vi "WPI_AccumulatorSetConfiguration.vi"(6 "Deadband":dbl, 8 "error in (no error)":errorcluster, 9 "Initial Value":dbl, 10 "Center":dbl, 11 "AIDeviceRef":T1={"DevStatus"={"status"=FALSE, "code"=0, "source"=""}, "Analog Channel"=enum."Invalid"}) -> (0 "error out":errorcluster, 3 "AIDeviceRef":T1={"DevStatus"={"status"=FALSE, "code"=0, "source"=""}, "Analog Channel"=enum."Invalid"})   [LabVIEW 2017]
doc: "Sets the center value, initial value, and deadband of the accumulator on the FPGA on the roboRIO device. The FPGA subtracts the center value from the value of each element before adding the value of the element to the cumulative value of the accumulator. Set the center value and initial value to account for offset in devices, such as gyros and accelerometers, when integrating signals from these devices. The accumulator does not accumulate a value if the difference between the center value and the current value is less than the deadband.\n\nThis software is licensed. Open the labview\\readme\\WPI Robotics Library Open Source License.txt file for more information."
uses:
  <vilib>/Rock Robotics/WPI/AnalogChannel/WPI_AnalogChannelDevRef.ctl
  <vilib>/Rock Robotics/SystemInterfaces/AI/FPGA_AIChannel.ctl
  <vilib>/Rock Robotics/SystemInterfaces/System/FPGA_SystemGet.vi
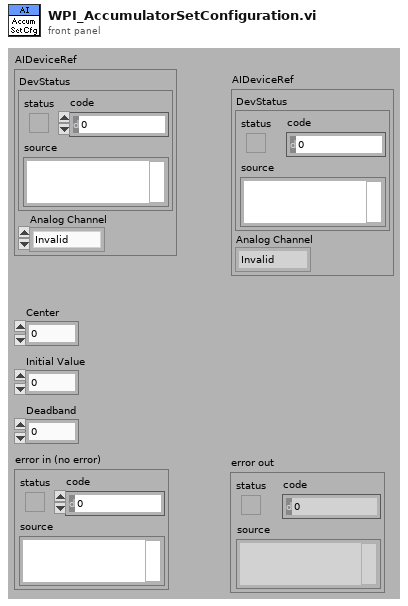
[diagram p1: front panel]
types:
  T1 = typedef "WPI_AnalogChannelDevRef.ctl" = cluster{"DevStatus":errorcluster, "Analog Channel":T2}
  T2 = typedef "FPGA_AIChannel.ctl" = enum8{"AI 0", "AI 1", "AI 2", "AI 3", "AI MXP 0", "AI MXP 1", "AI MXP 2", "AI MXP 3", "Invalid"}
  T3 = typedef "FPGA_AIDevRef.ctl" = cluster{"DevStatus":errorcluster}
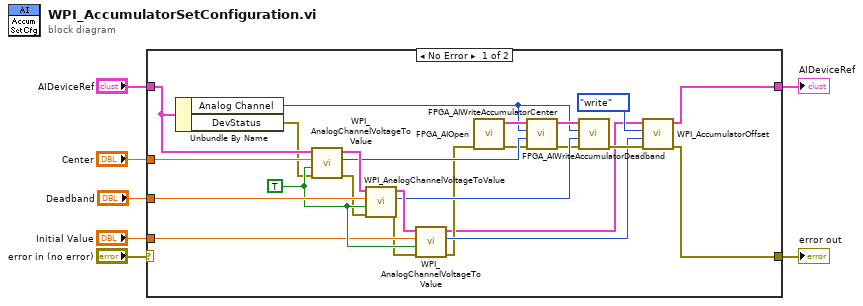
[diagram p0: block diagram]
diagram:
  n1 = case shown="No Error" "error in (no error)" {
    selector: "error in (no error)" -> [_ w32]
    tunnel: [w8 w33] -> w7
    tunnel: "AIDeviceRef" -> [w12 w33]
    tunnel: "Center" -> [w25 _]
    tunnel: [w29 w32] -> w3
    tunnel: "Initial Value" -> [w19 _]
    tunnel: "Deadband" -> [w21 _]
    frame No Error {
      w20 = TRUE ("Averaged")
      n2 = Unbundle By Name(w12) -> ("Analog Channel"=w26:T2, "DevStatus"=w10:errorcluster)
      n3 = call <vilib>:"WPI_AnalogChannelVoltageToValue.vi"("error in (no error)"=w10, "Averaged"=w20, "Voltage"=w25, "AIDeviceRef"=w12) -> ("error out"=w14:errorcluster, "Value"=w22:i32, "AIDeviceRef"=w24:T1)  [unwired: 1 in, 4 out]
      n4 = call <vilib>:"WPI_AnalogChannelVoltageToValue.vi"("error in (no error)"=w14, "Averaged"=w20, "Voltage"=w21, "AIDeviceRef"=w24) -> ("error out"=w13:errorcluster, "Value"=w18:i32, "AIDeviceRef"=w23:T1)  [unwired: 1 in, 4 out]
      n5 = call <vilib>:"WPI_AnalogChannelVoltageToValue.vi"("error in (no error)"=w13, "Averaged"=w20, "Voltage"=w19, "AIDeviceRef"=w23) -> ("error out"=w11:errorcluster, "Value"=w17:i32, "AIDeviceRef"=w9:T1)  [unwired: 1 in, 4 out]
      n6 = call <vilib>:"FPGA_AIOpen.vi"("error in (no error)"=w11) -> ("error out"=w16:errorcluster, "AI Reference out"=w31:T3)  [unwired: 2 in, 7 out]
      n7 = call <vilib>:"FPGA_AIWriteAccumulatorCenter.vi"("error in (no error)"=w16, "Center"=w22, "Channel"=w26, "AI Reference in"=w31) -> ("error out"=w15:errorcluster, "AI Reference out"=w28:T3)  [unwired: 6 out]
      n8 = call <vilib>:"FPGA_AIWriteAccumulatorDeadband.vi"("error in (no error)"=w15, "Deadband"=w18, "Channel"=w26, "AI Reference in"=w28) -> ("error out"=w27:errorcluster)  [unwired: 7 out]
      n9 = call <vilib>:"WPI_AccumulatorOffset.vi"("error in (no error)"=w27, "Offset In"=w17, "Action"=enum16{"read", "write"}."write" ("what do"), "AIDeviceRef"=w9) -> ("error out"=w29:errorcluster, "AIDeviceRef"=w8:T1)  [unwired: 6 out]
    }
    frame Error {
    }
  }
  "AIDeviceRef" <- w7
  "error out" <- w3
